vi "Get Width.vi"(8 "error in (no error)":errorcluster, 11 "Image in":refnum<class "Image.lvclass">) -> (0 "error out":errorcluster, 2 "Width":i32, 3 "Image out":refnum<class "Image.lvclass">)   [LabVIEW 2020, in "RPI.SenseHat.Display.lvlib" / "Image.lvclass"]
doc: "Returns the image width."
uses:
  Image.lvclass
  Image.lvclass/Image.ctl
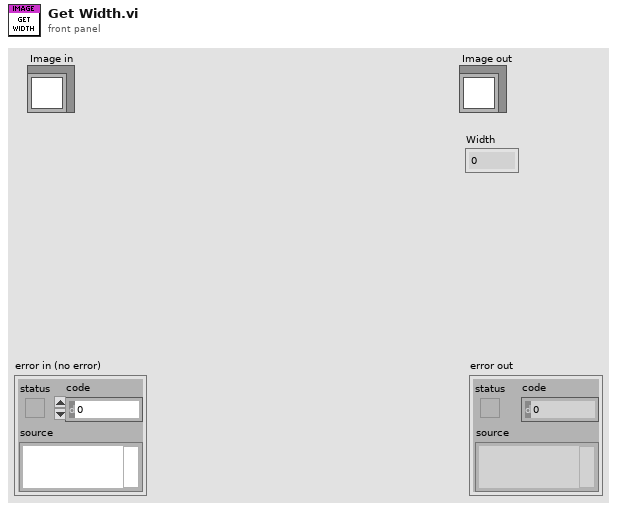
[diagram p1: front panel]
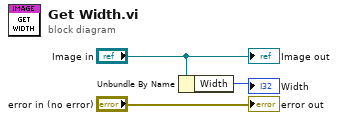
[diagram p0: block diagram]
diagram:
  n1 = Unbundle By Name("Image in") -> ("Width"=→"Width":i32)
  "error out" <- "error in (no error)"
  "Image out" <- "Image in"
